vi "List Modules(+SysLevel).vi"(8 "Error in":errorcluster caption="Error in (no error)") -> (0 "Error out":errorcluster, 3 "Module Names":string[](array[string]))   [LabVIEW 2017, in "Communicable State Machine.lvlib"]
doc: "List all active CSM modules.\n\n> [!NOTE] CSM Working Modes\n> 1. Stand-alone: Independent working mode. If no module name is provided, a random ID will be generated to identify the module.\n> 2. CSM: Regular CSM module.\n> 3. Action Worker: Worker mode. Add \"#\" after the module name to mark this module as a worker, sharing the same message queue with other workers of the same name.\n> 4. Chain Node: Chain node. Add \"$\" after the module name to mark this module as a chain node. Messages on the same chain will be passed sequentially until a node processes the message.\n\n\n-- <b>Controls</b> --\n- <b>Exclude Standalone CSM(T)</b>: Whether to include modules in standalone working mode\n\n-- <b>Indicators</b> --\n- <b>Module Names</b>: List of CSM module names"
uses:
  Communicable State Machine.lvlib
  CSMQ/_CSMOFGVOPER.ctl
  FGV-BroadcastRegistry/global-CSMQ FGV Change Flag.vi
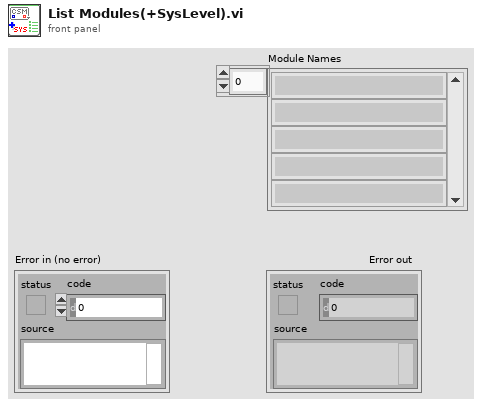
[diagram p1: front panel]
types:
  T1 = typedef "Communicable State Machine.lvlib/_CSMOFGVOPER.ctl" = enum16{"Create If not Exist", "Get By Name", "List", "Check If Name Exists", "Release", "Module Status", "Create Status Event Handler", "Destroy Status Event Handler"}
  T2 = typedef "Communicable State Machine.lvlib/_CSMObj.ctl" = cluster{"Requested Name":string, "Module Name":string, "Mode":T3, "Queue":refnum<class "Priority Queue.lvclass">, "CSM-Data":refnum<data-value>, "User Event":refnum<user-event>, "Status Change Event":refnum<user-event>, "Allowed Messages":string[], "Mode-Data":refnum<data-value>, "Group Name":string, "Exit Event":refnum<user-event>}
  T3 = typedef "Communicable State Machine.lvlib/_CSM_MODE.ctl" = enum16{"Not Exist", "Stand Alone", "CSM", "Worker Agent", "Worker", "Chain", "Chain Node"}
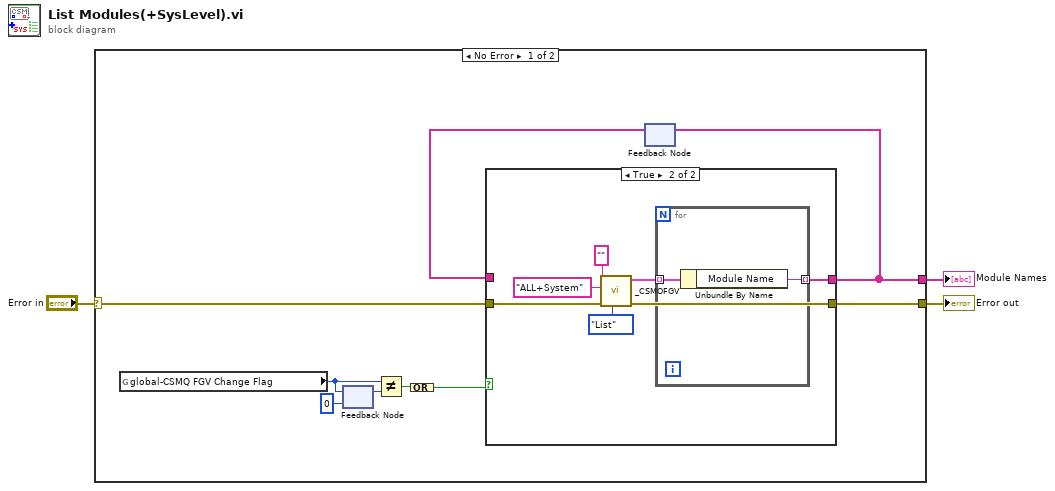
[diagram p0: block diagram]
diagram:
  n1 = case shown="No Error" "Error in" {
    selector: "Error in" -> [w12 w24]
    tunnel: [w11 w24] -> w2
    tunnel: [w4 _] -> w1
    frame No Error {
      n2 = global read "global-CSMQ FGV Change Flag.vi" "global-CSMQ FGV Change Flag"() -> (w9:u64)
      n3 = feedback #1(u64 0 ("global-CSMQ FGV Change Flag")) -> (w10:u64)
      n4 = feedback-in #1(w9) -> ()
      n5 = Not Equal?(x=w9, y=w10) -> (x != y?=w8:bool)
      n6 = Compound Arithmetic op=OR(w8) -> (w7:bool)
      n7 = feedback #2() -> (w6:string[])  [unwired: 1 in]
      n8 = case shown="True" w7 {
        tunnel: w12 -> [w14 w21]
        tunnel: [w14 w20] -> w11
        tunnel: [w13 w16] -> w4
        tunnel: w6 -> [w13 _]
        frame False {
        }
        frame True {
          n9 = call "_CSMOFGV.vi"("Operation"=_CSMOFGVOPER."List", "Error in"=w21, "Reference"="ALL+System", "Name(\"\" to use uuid) in"="" ("Name(\"\" to use uuid) in")) -> ("Error out"=w20:errorcluster, "Array"=w17:T2[])  [unwired: 5 in, 1 out]
          n10 = for {
            tunnel: w17 -> [w23] mode=indexing
            tunnel: [w22] -> w16 mode=indexing
            n11 = Unbundle By Name(w23) -> ("Module Name"=w22:string)
          }
        }
      }
      n12 = feedback-in #2(w4) -> ()
    }
    frame Error {
    }
  }
  "Error out" <- w2
  "Module Names" <- w1
